vi "Remove Nth Calibration Point.vi"(8 "error in (no error)":errorcluster, 9 "Nth Calibration Point":u32, 10 "Channel":T1, 11 "EPU452 in":refnum<class "EPU452.lvclass">) -> (0 "error out":errorcluster, 3 "EPU452 out":refnum<class "EPU452.lvclass">)   [LabVIEW 2018, in "EPU452.lvclass"]
uses:
  EPU452.lvclass
  Controls/Channels.ctl
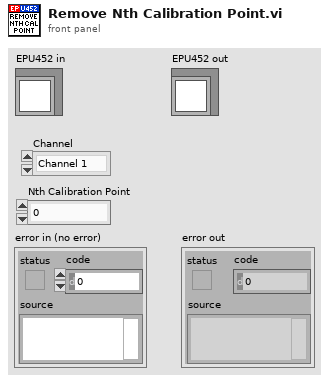
[diagram p1: front panel]
types:
  T1 = typedef "EPU452.lvclass/Channels.ctl" = enum16{"Channel 1", "Channel 2", "Channel 3", "Channel 4"}
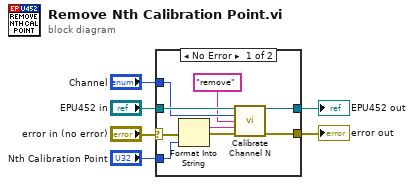
[diagram p0: block diagram]
diagram:
  n1 = case shown="No Error" "error in (no error)" {
    selector: "error in (no error)" -> [w10 w17]
    tunnel: [w12 w17] -> w5
    tunnel: [w13 w16] -> w3
    tunnel: "EPU452 in" -> [w15 w16]
    tunnel: "Channel" -> [w14 _]
    tunnel: "Nth Calibration Point" -> [w11 _]
    frame No Error {
      n2 = Format Into String(error in=w10, w11) -> (resulting string=w8:string, error out=w9:errorcluster)  [unwired: 2 in]
      n3 = call "Calibrate Channel N.vi"("EPU452 in"=w15, "Channel"=w14, "Function"="remove", "Argument/s"=w8, "error in (no error)"=w9) -> ("EPU452 out"=w13:refnum<class "EPU452.lvclass">, "error out"=w12:errorcluster)  [unwired: 8 in, 1 out]
    }
    frame Error {
    }
  }
  "error out" <- w5
  "EPU452 out" <- w3
